vi "Main.vi"() -> ()   [LabVIEW 2017]
uses:
  <vilib>/myRIO/Instrument Drivers/Onboard Devices/Accelerometer/typedefs/Accelerometer Reference.ctl
  <vilib>/myRIO/Common/Instrument Driver Framework/Utilities/typedefs/myRIO Generic Hardware Reference.ctl
  <vilib>/myRIO/Common/Instrument Driver Framework/Utilities/typedefs/Hardware Version Enum.ctl
  <vilib>/myRIO/Common/Instrument Driver Framework/Utilities/typedefs/myRIO v1.0 Reference.ctl
  <vilib>/myRIO/Common/Instrument Driver Framework/Utilities/typedefs/Generic FPGA Reference.ctl
  <vilib>/myRIO/Common/Instrument Driver Framework/myRIO v1.0/Accelerometer/typedefs/Accelerometer Channels List.ctl
  <vilib>/myRIO/Common/Instrument Driver Framework/myRIO v1.0/Accelerometer/typedefs/Accelerometer Channels Enum.ctl
  <vilib>/userdefined/High Color/nirio_resource_hc.ctl
  <vilib>/myRIO/Common/Instrument Driver Framework/Utilities/vis/Is FPGA Ref Available.vi
  <vilib>/myRIO/Common/Instrument Driver Framework/myRIO v1.0/Accelerometer/vis/myRIO v1.1 Open Accelerometer.vi
  <vilib>/myRIO/Instrument Drivers/Onboard Devices/Accelerometer/vis/Read.vi
  <vilib>/myRIO/Common/Instrument Driver Framework/Utilities/vis/Validate Channels.vi
  <vilib>/myRIO/Common/Instrument Driver Framework/myRIO v1.0/Accelerometer/vis/myRIO v1.0 Reserve Accelerometer.vi
  <vilib>/myRIO/Common/Instrument Driver Framework/myRIO v1.0/Resource Manager/vis/myRIO v1.0 Reserve Channel List.vi
  <vilib>/myRIO/Common/Instrument Driver Framework/myRIO v1.0/Accelerometer/vis/myRIO v1.0 Build MUX Configuration Accelerometer.vi
  <vilib>/myRIO/Common/Instrument Driver Framework/myRIO v1.0/Resource Manager/vis/myRIO v1.0 Reserve Channel.vi
  <vilib>/myRIO/Common/Instrument Driver Framework/myRIO v1.0/Resource Manager/vis/myRIO v1.0 Unreserve Channel.vi
  <vilib>/myRIO/Common/Instrument Driver Framework/myRIO v1.0/Resource Manager/vis/myRIO v1.0 Build Mutex Name.vi
  <vilib>/Instr/_visa.llb/VISA Configure Serial Port (Instr).vi
  <vilib>/addons/control/pid/pid.llb/PID (DBL).vi
  <vilib>/Utility/VariantDataType/GetNumericInfo.vi
  <vilib>/Utility/error.llb/Error Cluster From Error Code.vi
  <vilib>/myRIO/Common/Instrument Driver Framework/myRIO v1.0/myRIO v1.1 Open.vi
  <vilib>/myRIO/Common/Instrument Driver Framework/myRIO v1.0/Accelerometer/vis/myRIO v1.0 Get Scaling Constant Accelerometer.vi
  <vilib>/myRIO/Common/Instrument Driver Framework/Utilities/vis/IO Manager.vi
  <vilib>/myRIO/Common/Instrument Driver Framework/Utilities/vis/Configuration Manager.vi
  <vilib>/myRIO/Common/Instrument Driver Framework/myRIO v1.0/myRIO v1.0 Close.vi
  <vilib>/myRIO/Common/Instrument Driver Framework/myRIO v1.0/Accelerometer/vis/myRIO v1.0 Read Accelerometer.vi
  <vilib>/myRIO/Express VI/Onboard Devices/Accelerometer/Accelerometer Express VI.xnode
  <vilib>/myRIO/Instrument Drivers/Onboard Devices/Accelerometer/vis/myRIO Accelerometer Open.xnode
  <vilib>/addons/control/pid/NI_PID_pid.lvlib
  <vilib>/myRIO/Instrument Drivers/Onboard Devices/Accelerometer/Accelerometer.lvlib
panel:
  in  "Servo pulse width in mS":dbl(slide) scale=1.2..1.7
  out "ENCODER A":dbl
  out "ENCODER B":dbl
  in  "Boolean":bool
  out "Wheel A Direction 2":bool
  out "Wheel A Direction 1":bool
  out "PID Output 2":dbl(graph)
  in  "Numeric 2":i32
  in  "PID gains 2":T1={"proportional gain (Kc)"=1.0, "integral time (Ti, min)"=0.01, "derivative time (Td, min)"=0.0} {"derivative time (Td, min)" format="%.3f"; "integral time (Ti, min)" format="%.3f"; "proportional gain (Kc)" format="%.3f"}
  out "Accelerometer ranged":dbl(graph)
  out "Roll":dbl(graph)
  out "PID":cluster{dbl, "error":dbl, "setpoint":dbl}(graph)
  out "PID Output":dbl(graph)
  in  "Numeric":i32
  out "Wheel A PWM":dbl format="%.2f"
  in  "setpoint":dbl format="%.2f"
  in  "PID gains":T1={"proportional gain (Kc)"=1.0, "integral time (Ti, min)"=0.01, "derivative time (Td, min)"=0.0} {"derivative time (Td, min)" format="%.3f"; "integral time (Ti, min)" format="%.3f"; "proportional gain (Kc)" format="%.3f"}
  in  "Button":bool
  out "Roll":dbl
  out "Yaw":dbl
  out "read buffer":string
  in  "VISA resource name":refnum<visa-resource-name>
  out "Waveform Chart":cluster{dbl, dbl, dbl}(graph)
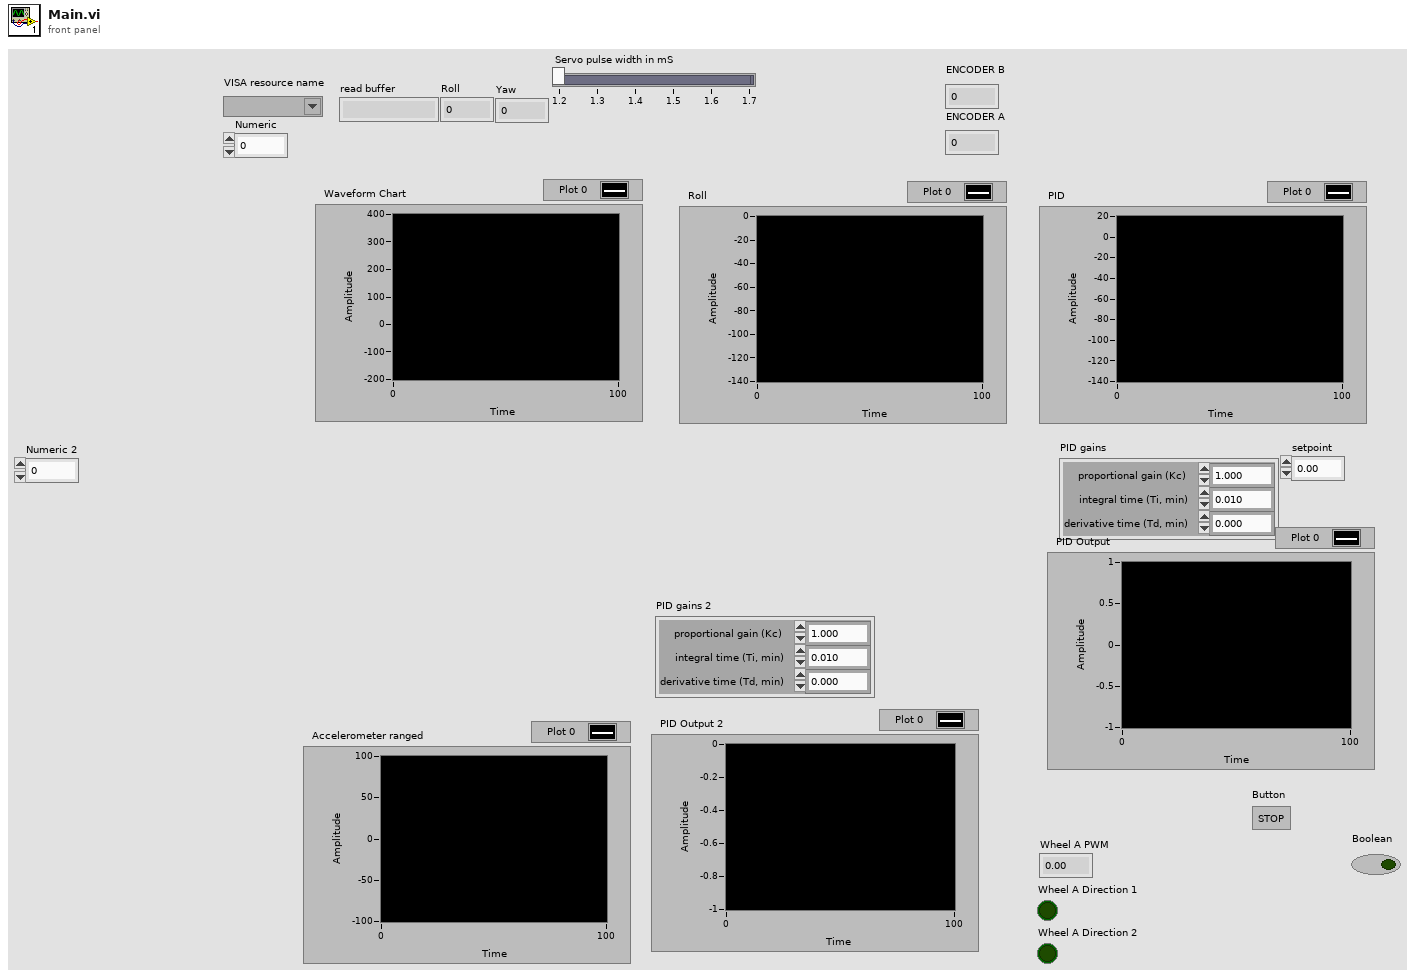
[diagram p1: front panel]
types:
  T1 = cluster{"proportional gain (Kc)":dbl, "integral time (Ti, min)":dbl, "derivative time (Td, min)":dbl}
  T2 = typedef "Accelerometer.lvlib/Accelerometer Reference.ctl" = cluster{"myRIO Reference":T3, "Accelerometer Channels List":T7, "LSB Weight":dbl}
  T3 = typedef "myRIO Generic Hardware Reference.ctl" = cluster{"myRIO Model":T4, "myRIO Hardware Reference":T5}
  T4 = typedef "Hardware Version Enum.ctl" = enum16{"Unknown", "myRIO-1900", "myRIO-1950", "roboRIO", "NI ELVIS RIO CM"}
  T5 = typedef "myRIO v1.0 Reference.ctl" = cluster{"Generic FPGA Reference":T6, "Allow multiple opens":bool}
  T6 = typedef "Generic FPGA Reference.ctl" = refnum<k20>
  T7 = typedef "Accelerometer Channels List.ctl" = T8[]
  T8 = typedef "Accelerometer Channels Enum.ctl" = enum16{"Not Connected", "X-Axis", "Y-Axis", "Z-Axis"}
  T9 = typedef "nirio_resource_hc.ctl" = tag
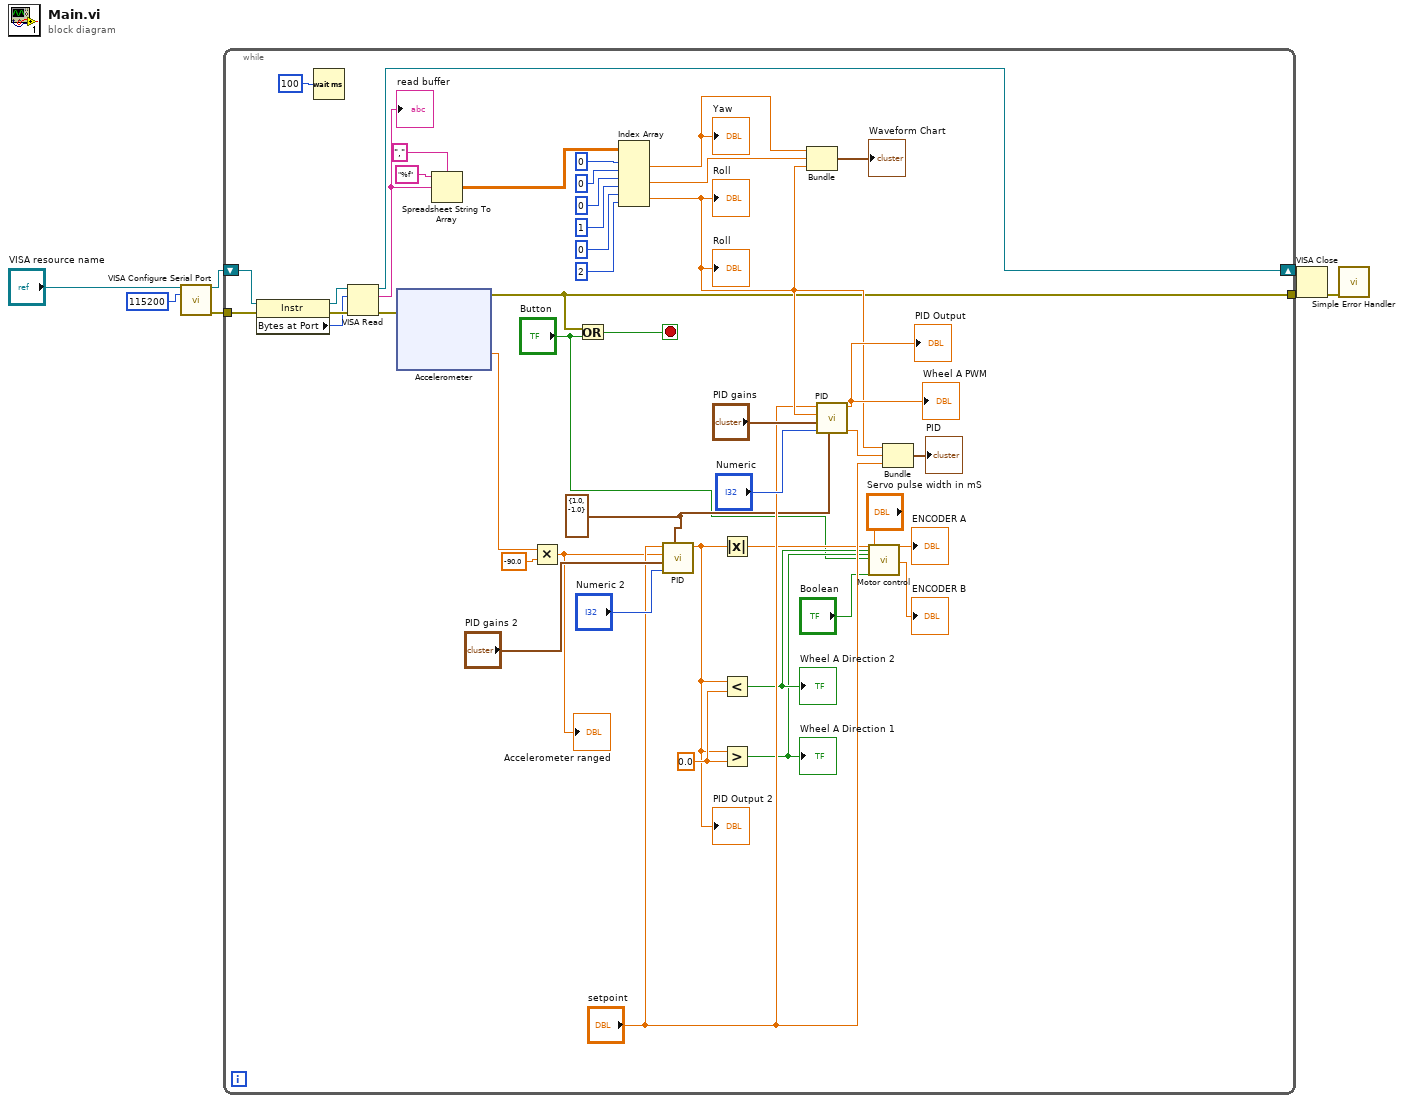
[diagram p0: block diagram]
diagram:
  n1 = call-poly "VISA Configure Serial Port"("VISA resource name"="VISA resource name", "baud rate (9600)"=u32 115200 ("baud rate")) -> ("VISA resource name out"=w5:refnum<visa-resource-name>, "error out"=w4:errorcluster)  [unwired: 12 in]
  n2 = while {
    tunnel: w4 -> [w52]
    shift-right: [w36] -> w2
    shift-left: w5 -> [w53]
    tunnel: [w12] -> w1
    stop <- w37 stop-if-true
    w18 = 0.0 ("y")
    w19 = cluster{"output high":dbl, "output low":dbl} {"output high"=1.0, "output low"=-1.0} ("output range")
    n3 = property class="Instr"(reference=w53, error in=w52) -> (reference out=w51:refnum<visa-resource-name>, error out=w50:errorcluster, "Bytes at Port"=w49:u32)
    n4 = Wait (ms)(milliseconds to wait=u32 100) -> ()  [unwired: 1 out]
    n5 = VISA Read(VISA resource name=w51, byte count=w49, error in (no error)=w50) -> (VISA resource name out=w36:refnum<visa-resource-name>, read buffer=w46:string, error out=w27:errorcluster)  [unwired: 1 out]
    "read buffer" <- w46
    n6 = xnode "Accelerometer"("error in (no error)"=w27) -> ("X-Axis"=w24:dbl, "error out"=w12:errorcluster)  [unwired: 2 out]
    n7 = Spreadsheet String To Array(delimiter (Tab)=",", format string="%f", spreadsheet string=w46) -> (array=w45:dbl[][])  [unwired: 1 in]
    n8 = Multiply(x=w24, y=-90.0) -> (x*y=w20:dbl)
    "Accelerometer ranged" <- w20
    n9 = Or(x=w12, y="Button") -> (x .or. y?=w37:bool)
    n10 = Index Array(array=w45, index (row) #1=0 ("index (row)"), index (col) #1=0 ("disabled index (col)"), index (row) #2=0 ("index (row)"), index (col) #2=1 ("disabled index (col)"), index (row) #3=0 ("index (row)"), index (col) #3=2 ("disabled index (col)")) -> (element #1=w35:dbl, element #2=w30:dbl, element #3=w26:dbl)
    "Yaw" <- w35
    "Roll" <- w26
    "Roll" <- w26
    n11 = call-poly <vilib>:"PID.vi"("output range"=w19, "dt (s)"="Numeric 2", "PID gains"="PID gains 2", "process variable"=w20, "setpoint"="setpoint") -> ("output"=w17:dbl)  [unwired: 5 in, 1 out]
    "PID Output 2" <- w17
    n12 = Absolute Value(x=w17) -> (abs(x)=w16:dbl)
    n13 = Less?(x=w17, y=w18) -> (x < y?=w15:bool)
    "Wheel A Direction 2" <- w15
    n14 = Greater?(x=w17, y=w18) -> (0:w14:bool)
    "Wheel A Direction 1" <- w14
    n15 = Bundle(w35, w30, w26) -> (→"Waveform Chart":cluster{dbl, dbl, dbl})  [unwired: 1 in]
    n16 = call-poly <vilib>:"PID.vi"("output range"=w19, "dt (s)"="Numeric", "PID gains"="PID gains", "process variable"=w26, "setpoint"="setpoint") -> ("dt out (s)"=w29:dbl, "output"=→"Wheel A PWM" →"PID Output":dbl)  [unwired: 5 in]
    n17 = call "Motor control.vi"("PWM   DIO8"=w16, "DIR1 DIO4"=w15, "DIR2 DIO5"=w14, "Stop"="Button", "Standby B/DIO7 (Pin 25)"="Boolean", "Servo pulse width in mS"="Servo pulse width in mS") -> ("ENCODER A"=→"ENCODER A":dbl, "ENCODER B"=→"ENCODER B":dbl)  [unwired: 20 in]
    n18 = Bundle(w26, "dt out (s)"=w29, "setpoint"="setpoint") -> (→"PID":cluster{dbl, "dt out (s)":dbl, "setpoint":dbl})  [unwired: 1 in]
  }
  n19 = VISA Close(VISA resource name=w2, error in (no error)=w1) -> (error out=w3:errorcluster)
  n20 = call <vilib>:"Simple Error Handler.vi"("error in (no error)"=w3) -> ()  [unwired: 4 in, 5 out]
